vi "Pass If Approved.vi"(8 "error in (no error)":errorcluster, 11 "Test Data":string) -> (0 "error out":errorcluster, 2 "Failure Message":string, 3 "Passed?":bool)   [LabVIEW 2020]
doc: "Performs an approval test.\n\nThe first call, the test passes and the test data is written to the approved file.\n\nOn subsequent runs the test data is compared to the contents of the approved file.\nIf it is a match, the test passes.\nIf it is not a match, the test fails and the test data is written to the actual file.\n\nAt the point the user can diff the approved and actual files and determine if they approve of the changes or not. If they approve, they replace the old approved file with the actual file. \n\nNOTE: You should keep the approved files in Source Code Control. You should ignore *.actual in your .gitignore file - there is no need to store those."
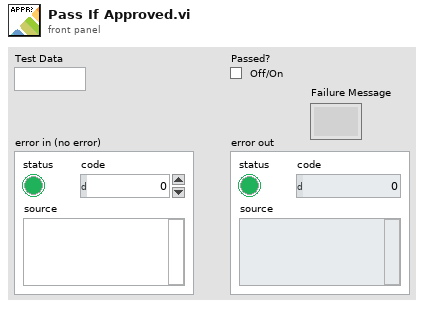
[diagram p1: front panel]
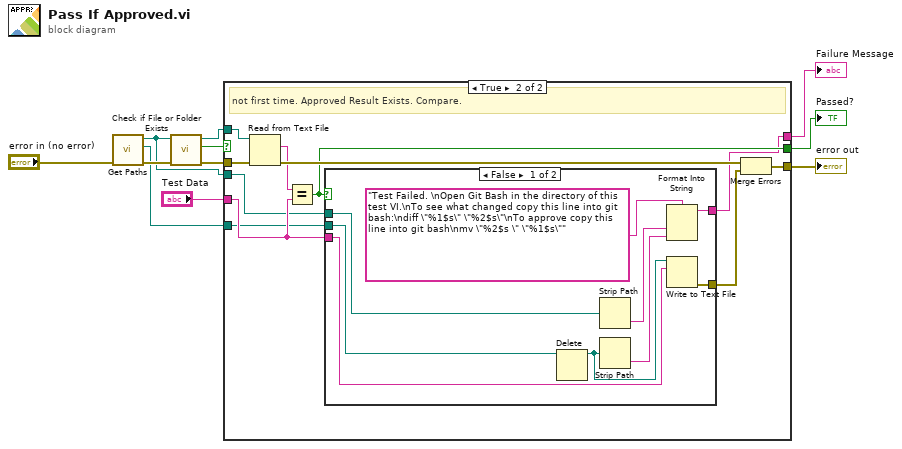
[diagram p0: block diagram]
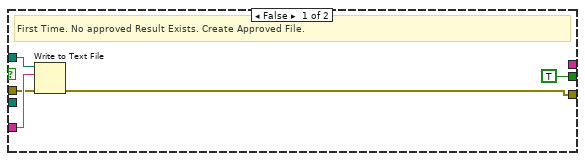
[diagram p2: hidden frame]
diagram:
  n1 = call "Get Paths.vi"("error in (no error)"="error in (no error)") -> ("error out"=w8:errorcluster, "actual path"=w3:path, "approved path"=w1:path)  [unwired: 8 in]
  n2 = call <vilib>:"Check if File or Folder Exists.vi"("error in (no error)"=w8, "path"=w1) -> ("error out"=w7:errorcluster, "file or folder exists?"=w5:bool, "dup path"=w6:path)  [unwired: 7 in]
  n3 = case shown="True" w5 {
    tunnel: "Test Data" -> [w16 w22]
    tunnel: [w15 w20] -> w10
    tunnel: w7 -> [w14 w27]
    tunnel: w6 -> [w13 w25]
    tunnel: [TRUE ("Passed?") w23] -> w4
    tunnel: w3 -> [_ w21]
    tunnel: [_ w18] -> w2
    tunnel: w1 -> [_ w17]
    frame False {
      # "First Time. No approved Result Exists. Create Approved File."
      n4 = Write to Text File(file (use dialog)=w13, text=w16, error in=w14) -> (error out=w15:errorcluster)  [unwired: 1 in, 2 out]
    }
    frame True {
      # "not first time. Approved Result Exists. Compare."
      n5 = Read from Text File(file (use dialog)=w25, error in=w27) -> (text=w24:string, error out=w26:errorcluster)  [unwired: 2 in, 2 out]
      n6 = Equal?(x=w24, y=w22) -> (x = y?=w23:bool)
      n7 = case shown="False" w23 {
        tunnel: w22 -> [w35 _]
        tunnel: w21 -> [w36 _]
        tunnel: [w34 _] -> w19
        tunnel: [w33 _] -> w18
        tunnel: w17 -> [w29 _]
        frame False {
          n8 = Delete(path (use dialog)=w36) -> (deleted path=w28:path)  [unwired: 4 in, 2 out]
          n9 = Strip Path(path=w29) -> (name=w31:string)  [unwired: 1 out]
          n10 = Strip Path(path=w28) -> (name=w30:string)  [unwired: 1 out]
          n11 = Format Into String(format string="Test Failed. \nOpen Git Bash in the directory of this test VI.\nTo see what changed copy this line into git bash:\ndiff \"%1$s\" \"%2$s\"\nTo approve copy this line into git bash\nmv \"%2$s \" \"%1$s\"", w31, w30) -> (resulting string=w33:string)  [unwired: 2 in, 1 out]
          n12 = Write to Text File(file (use dialog)=w28, text=w35) -> (error out=w34:errorcluster)  [unwired: 2 in, 2 out]
        }
        frame True {
        }
      }
      n13 = Merge Errors(w26, w19) -> (w20:errorcluster)
    }
  }
  "error out" <- w10
  "Passed?" <- w4
  "Failure Message" <- w2
